vi "SeCrTs-Data Transfer Loop.vi"(9 "Message Queue 2":refnum<queue>, 11 "Data FIFO Ref":T1) -> ()   [LabVIEW 2022 SP3]
uses:
  RT Support/RT_Global_R.vi
  RT Controls/DiplayPC comm ctrl.ctl
  RT Controls/Message Cluster_R.ctl
  RT Controls/Data FIFO.ctl
panel:
  out "x-y":u32
  in  "Message Queue":refnum<queue>
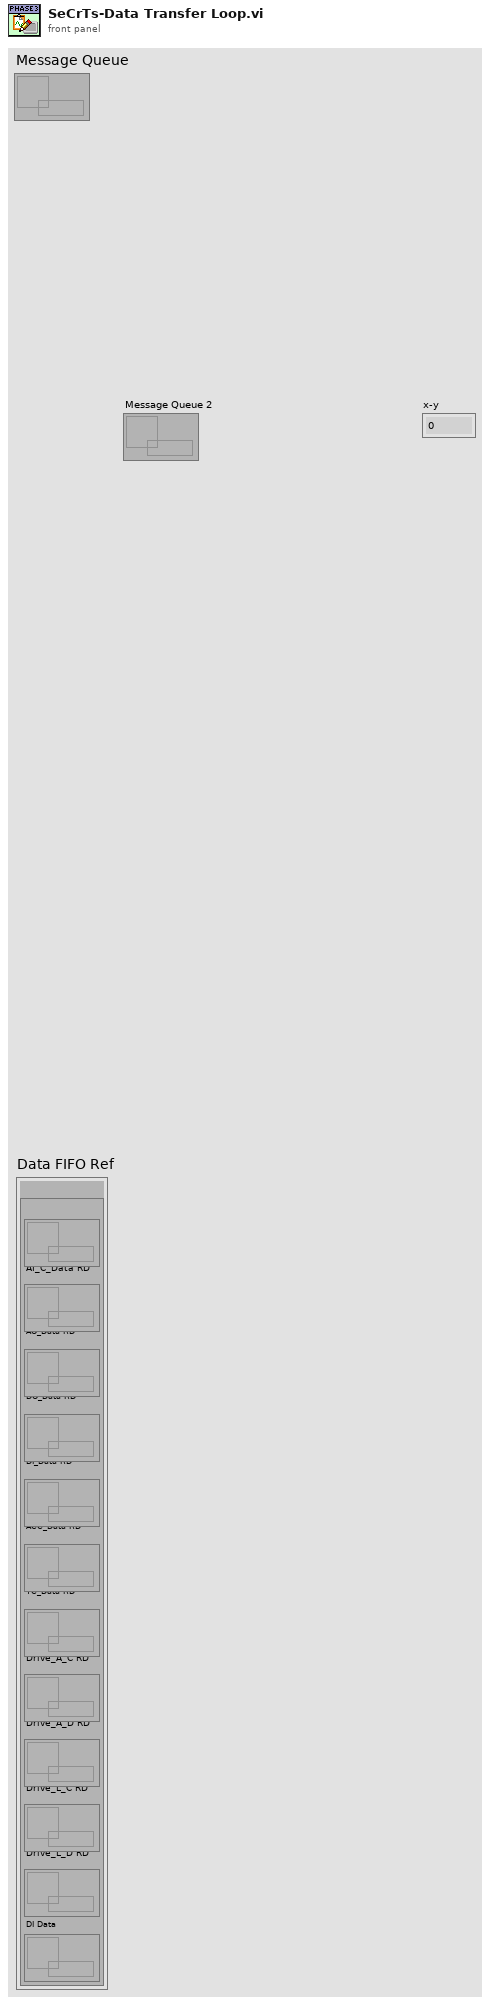
[diagram p1: front panel]
types:
  T1 = typedef "Data FIFO.ctl" = cluster{"RD":cluster{"AI_V_Data RD":refnum<queue>, "AI_C_Data RD":refnum<queue>, "AO_Data RD":refnum<queue>, "DO_Data RD":refnum<queue>, "DI_Data RD":refnum<queue>, "ACC_Data RD":refnum<queue>, "TC_Data RD":refnum<queue>, "Drive_A_C RD":refnum<queue>, "Drive_A_D RD":refnum<queue>, "Drive_L_C RD":refnum<queue>, "Drive_L_D RD":refnum<queue>, "DI Data":refnum<queue>}}
  T2 = typedef "DiplayPC comm ctrl.ctl" = enum16{"Initialize", "Listen for UI Writer", "Send RT Data"}
  T3 = cluster{"AI_V_Data":waveform(dbl)[][], "AI_C_Data":waveform(dbl)[], "AO_Data":waveform(dbl)[], "DO_Data":waveform(dbl)[], "DI_Data":digitalwaveform[][], "ACC_Data":waveform(dbl)[], "TC Data":waveform(dbl)[], "Drive_A_C":waveform(dbl)[], "Drive_A_D":waveform(dbl)[], "Drive_L_C":waveform(dbl)[], "Drive_L_D":waveform(dbl)[]}
  T4 = cluster{"Start DAQ":bool, "Stop DAQ":bool, "RT Stop":bool, "RT Exit":bool, "Start Seq":bool}
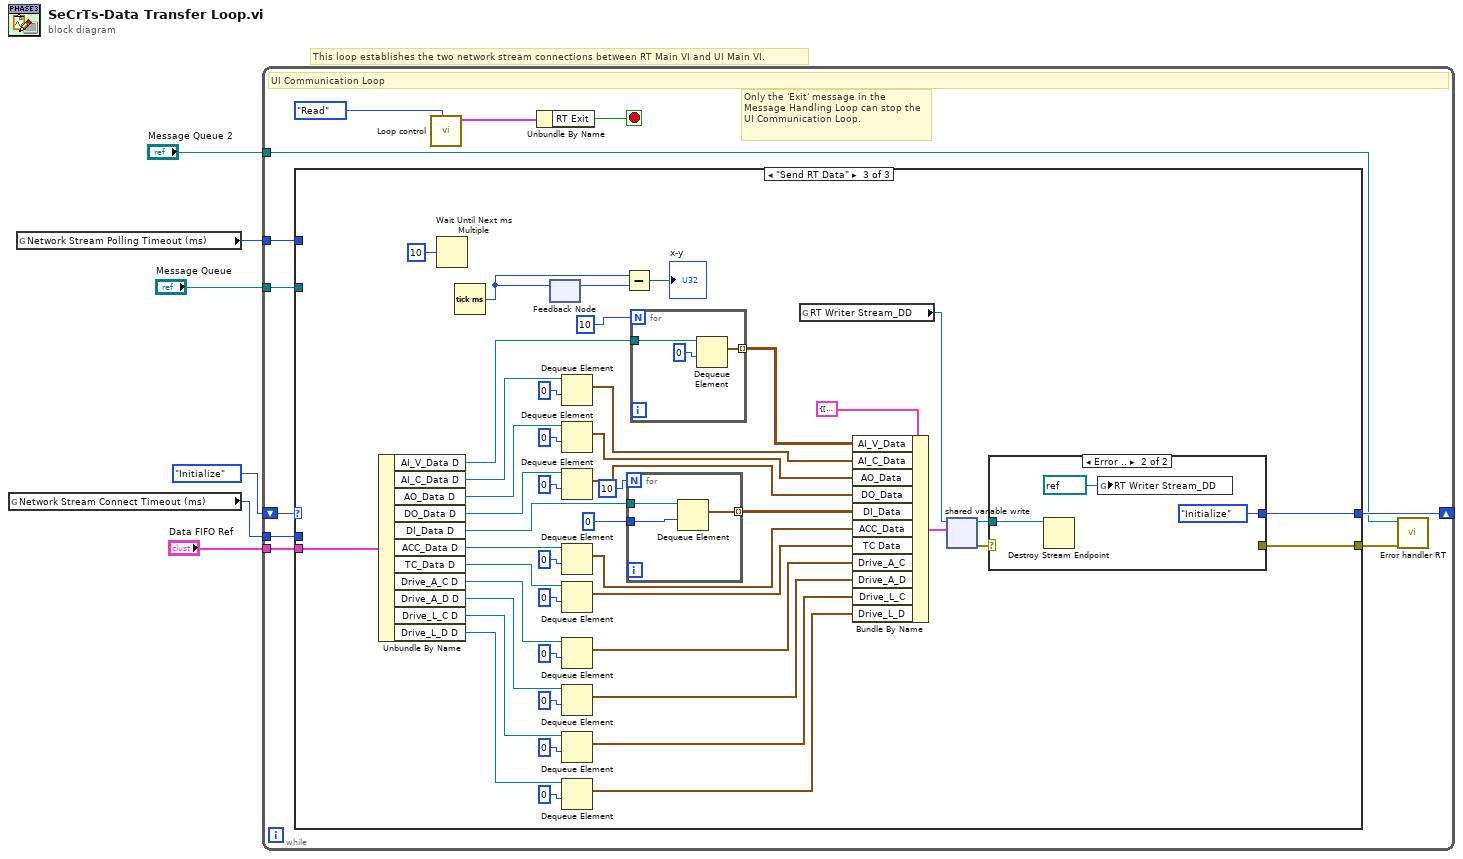
[diagram p0: block diagram]
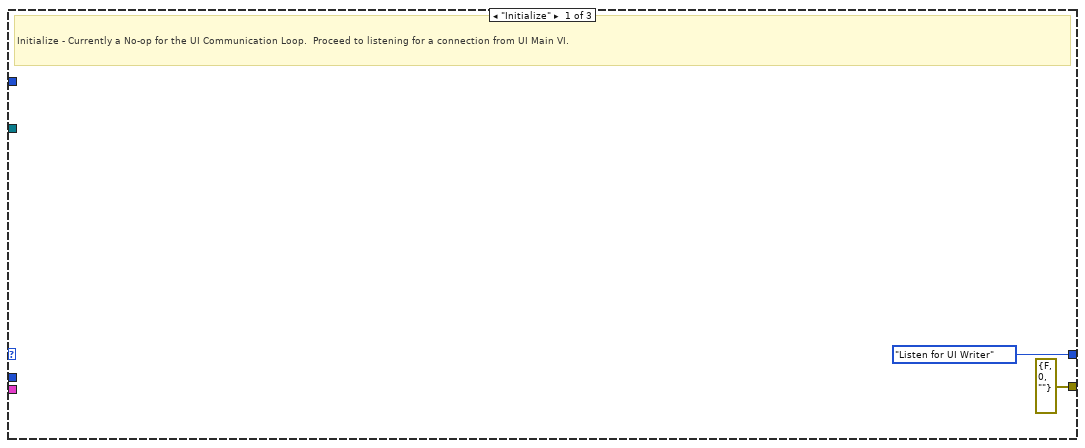
[diagram p2: hidden frame]
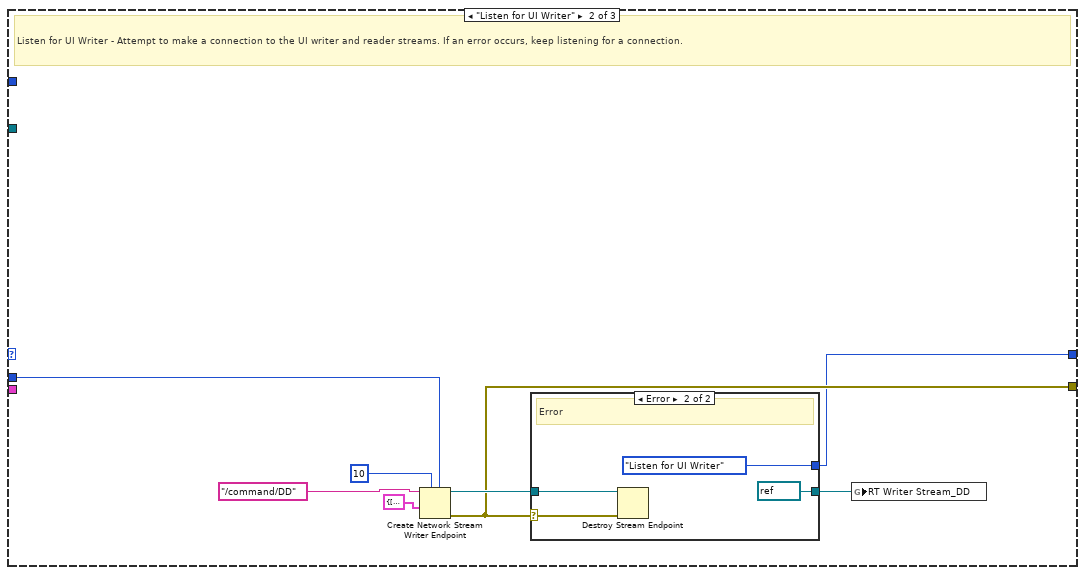
[diagram p3: hidden frame]
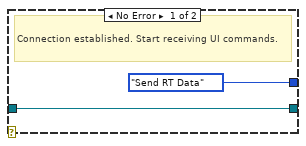
[diagram p4: hidden frame]
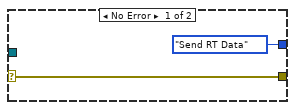
[diagram p5: hidden frame]
diagram:
  # "This loop establishes the two network stream connections between RT Main VI and UI Main VI."
  n1 = global read "RT_Global_R.vi" "Network Stream Connect Timeout (ms)"() -> (w4:i32)
  n2 = global read "RT_Global_R.vi" "Network Stream Polling Timeout (ms)"() -> (w5:i32)
  n3 = while {
    tunnel: "Message Queue" -> [w14]
    tunnel: w5 -> [w17]
    tunnel: w4 -> [w16]
    shift-right: [w15] -> _
    shift-left: DiplayPC_comm_ctrl."Initialize" -> [w13]
    tunnel: "Data FIFO Ref" -> [w12]
    tunnel: "Message Queue 2" -> [w7]
    stop <- w9 stop-if-true
    # "Only the 'Exit' message in the  Message Handling Loop can stop the UI Communication Loop."
    # "UI Communication Loop"
    n4 = case shown="\"Send RT Data\"" w13 {
      tunnel: [errorcluster {"status"=FALSE, "code"=0, "source"=""} ("error IO") w26 w78] -> w8
      tunnel: w16 -> [_ w25 _]
      tunnel: w14 -> [_ _ _]
      tunnel: w17 -> [_ _ _]
      tunnel: [DiplayPC_comm_ctrl."Listen for UI Writer" w23 w52] -> w15
      tunnel: w12 -> [_ _ w75]
      frame "Initialize" {
        # "Initialize - Currently a No-op for the UI Communication Loop.  Proceed to listening for a connection from UI Main VI."
      }
      frame "Listen for UI Writer" {
        # "Listen for UI Writer - Attempt to make a connection to the UI writer and reader streams. If an error occurs, keep listening for a connection."
        n5 = Create Network Stream Writer Endpoint(5:w25, 7:10 ("writer buffer size"), 9:T3 {"AI_V_Data"=[], "AI_C_Data"=[], "AO_Data"=[], "DO_Data"=[], "DI_Data"=[], "ACC_Data"=[], "TC Data"=[], "Drive_A_C"=[], "Drive_A_D"=[], "Drive_L_C"=[], "Drive_L_D"=[]}, 11:"/command/DD" ("reader url")) -> (0:w26:errorcluster, 3:w27:refnum<k21>)  [unwired: 3 in]
        n6 = case shown="Error" w26 {
          selector: w26 -> [_ w31]
          tunnel: w27 -> [w28 w33]
          tunnel: [DiplayPC_comm_ctrl."Send RT Data" DiplayPC_comm_ctrl."Listen for UI Writer"] -> w23
          tunnel: [w28 refnum<k21> refnum ("reader url")] -> w22
          frame No Error {
            # "Connection established. Start receiving UI commands."
          }
          frame Error {
            # "Error"
            n7 = Destroy Stream Endpoint(8:w31, 11:w33) -> ()  [unwired: 1 out]
          }
        }
        n8 = global write "RT_Global_R.vi" "RT Writer Stream_DD"(w22) -> ()
      }
      frame "Send RT Data" {
        n9 = Unbundle By Name(w75) -> ("AI_V_Data D"=w74:refnum<queue>, "AI_C_Data D"=w73:refnum<queue>, "AO_Data D"=w72:refnum<queue>, "DO_Data D"=w71:refnum<queue>, "DI_Data D"=w70:refnum<queue>, "ACC_Data D"=w69:refnum<queue>, "TC_Data D"=w68:refnum<queue>, "Drive_A_C D"=w67:refnum<queue>, "Drive_A_D D"=w66:refnum<queue>, "Drive_L_C D"=w65:refnum<queue>, "Drive_L_D D"=w64:refnum<queue>)
        n10 = Wait Until Next ms Multiple(millisecond multiple=u32 10) -> ()  [unwired: 1 out]
        n11 = Tick Count (ms)() -> (millisecond timer value=w41:u32)
        n12 = feedback-in #1(w41) -> ()
        n13 = feedback #1() -> (w40:u32)  [unwired: 1 in]
        n14 = Dequeue Element(queue=w73, timeout in ms (-1)=0) -> (element=w54:waveform(dbl)[])  [unwired: 1 in, 3 out]
        n15 = Dequeue Element(queue=w72, timeout in ms (-1)=0) -> (element=w62:waveform(dbl)[])  [unwired: 1 in, 3 out]
        n16 = Dequeue Element(queue=w71, timeout in ms (-1)=0) -> (element=w61:waveform(dbl)[])  [unwired: 1 in, 3 out]
        n17 = Dequeue Element(queue=w69, timeout in ms (-1)=0) -> (element=w59:waveform(dbl)[])  [unwired: 1 in, 3 out]
        n18 = Dequeue Element(queue=w68, timeout in ms (-1)=0) -> (element=w58:waveform(dbl)[])  [unwired: 1 in, 3 out]
        n19 = Dequeue Element(queue=w67, timeout in ms (-1)=0) -> (element=w57:waveform(dbl)[])  [unwired: 1 in, 3 out]
        n20 = Dequeue Element(queue=w66, timeout in ms (-1)=0) -> (element=w56:waveform(dbl)[])  [unwired: 1 in, 3 out]
        n21 = Dequeue Element(queue=w65, timeout in ms (-1)=0) -> (element=w55:waveform(dbl)[])  [unwired: 1 in, 3 out]
        n22 = Dequeue Element(queue=w64, timeout in ms (-1)=0) -> (element=w53:waveform(dbl)[])  [unwired: 1 in, 3 out]
        n23 = Subtract(x=w41, y=w40) -> (x-y=→"x-y":u32)
        n24 = for {
          N: 10 -> [_]
          tunnel: w70 -> [w82]
          tunnel: [w81] -> w60 mode=indexing
          tunnel: 0 ("timeout in ms (-1)") -> [w80]
          n25 = Dequeue Element(queue=w82, timeout in ms (-1)=w80) -> (element=w81:digitalwaveform[])  [unwired: 1 in, 3 out]
        }
        n26 = for {
          N: 10 -> [_]
          tunnel: w74 -> [w85]
          tunnel: [w84] -> w63 mode=indexing
          n27 = Dequeue Element(queue=w85, timeout in ms (-1)=0) -> (element=w84:waveform(dbl)[])  [unwired: 1 in, 3 out]
        }
        n28 = global read "RT_Global_R.vi" "RT Writer Stream_DD"() -> (w76:refnum<k21>)
        n29 = Bundle By Name(cluster=T3 {"AI_V_Data"=[], "AI_C_Data"=[], "AO_Data"=[], "DO_Data"=[], "DI_Data"=[], "ACC_Data"=[], "TC Data"=[], "Drive_A_C"=[], "Drive_A_D"=[], "Drive_L_C"=[], "Drive_L_D"=[]}, "AI_V_Data"=w63, "AI_C_Data"=w54, "AO_Data"=w62, "DO_Data"=w61, "DI_Data"=w60, "ACC_Data"=w59, "TC Data"=w58, "Drive_A_C"=w57, "Drive_A_D"=w56, "Drive_L_C"=w55, "Drive_L_D"=w53) -> (w38:T3)
        n30 = shared-variable-write(w76, w38) -> (w77:refnum<k21>, w79:errorcluster)  [unwired: 2 in, 1 out]
        n31 = case shown="Error .." w79 {
          selector: w79 -> [w87 _]
          tunnel: [w87 _] -> w78
          tunnel: w77 -> [_ w90]
          tunnel: [DiplayPC_comm_ctrl."Send RT Data" DiplayPC_comm_ctrl."Initialize"] -> w52
          frame No Error {
          }
          frame Error {
            n32 = Destroy Stream Endpoint(11:w90) -> ()  [unwired: 1 in, 1 out]
            n33 = global write "RT_Global_R.vi" "RT Writer Stream_DD"(refnum<k21> refnum ("RT Writer Stream_DD")) -> ()
          }
        }
      }
    }
    n34 = call "Loop control.vi"("Action"=enum16{"Init", "Write", "Read"}."Read") -> ("Loop Control out"=w11:T4)  [unwired: 9 in, 1 out]
    n35 = Unbundle By Name(w11) -> ("RT Exit"=w9:bool)
    n36 = call "Error handler RT.vi"("error in"=w8, "Message Queue"=w7) -> ()  [unwired: 8 in, 2 out]
  }
